vi "test-FIX Helper Dialog.vi"() -> ()   [LabVIEW 2017]
panel:
  in  "Bottom Text":string="Communicable State Machine(CSM) v2024.11.28.152636        "
  out "2D Picture":picture
  out "Progress Bar":i32(slide) scale=0.0..100.0
  in  "path to PNG file":path
  # "图片尺寸=768 x 432"
  # "VI 宽度=768-24=744"
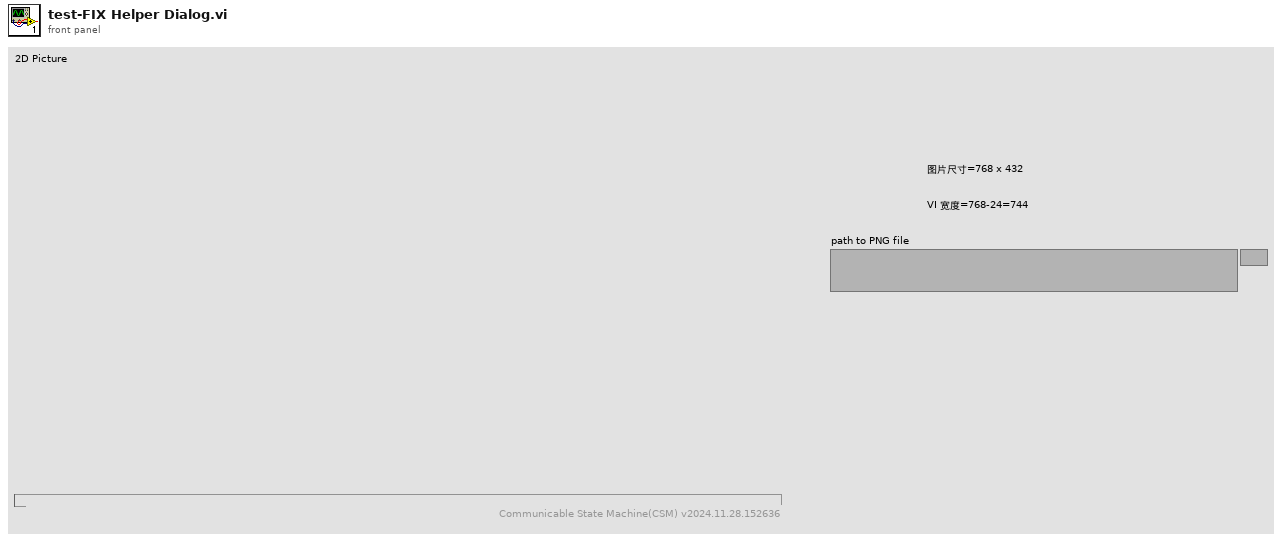
[diagram p1: front panel]
types:
  T1 = typedef "imagedata.ctl" = cluster{"image type":i32, "image depth":i32, "image":u8[], "mask":u8[], "colors":u32[], "Rectangle":cluster{"left":i16, "top":i16, "right":i16, "bottom":i16}}
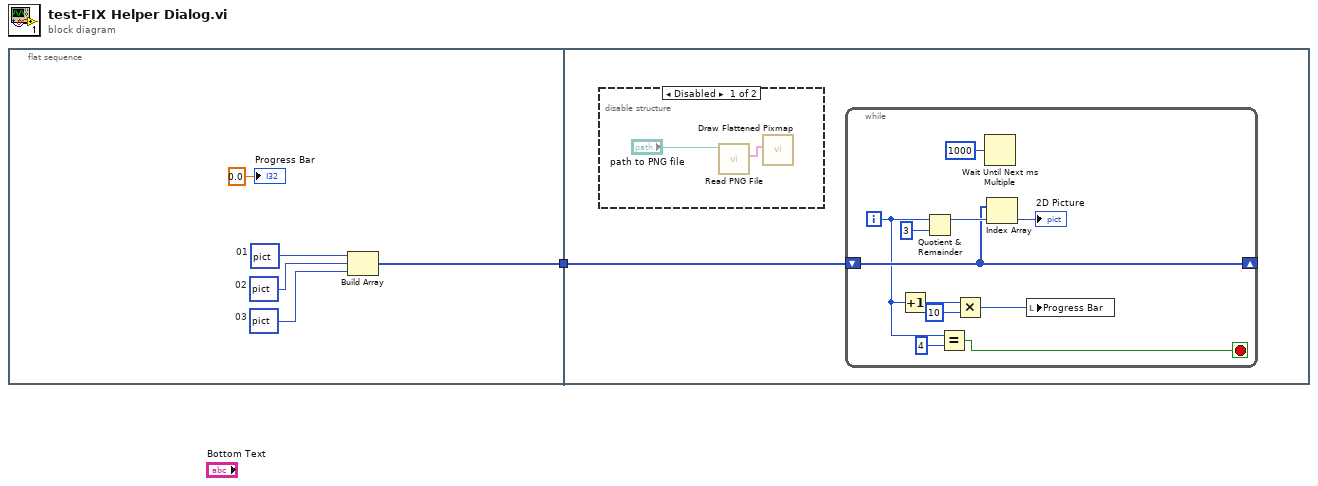
[diagram p0: block diagram]
diagram:
  n1 = flat-sequence {
    tunnel: [w3] -> w1
    tunnel: w1 -> [w7]
    frame #0 {
      w4 = picture bytes[1036830]  # 03
      w5 = picture bytes[1036830]  # 02
      w6 = picture bytes[1036830]  # 01
      n2 = Build Array(w6, w5, w4) -> (w3:picture[])
      "Progress Bar" <- 0.0 ("Progress Bar")
    }
    frame #1 {
      n3 = disable-structure shown="Disabled" {
        frame Disabled {
          n4 = call <vilib>:"Read PNG File.vi"("path to PNG file"="path to PNG file") -> ("image data"=w20:T1)  [unwired: 8 in, 2 out]
          n5 = call <vilib>:"Draw Flattened Pixmap.vi"("image data"=w20) -> ()  [unwired: 8 in, 1 out]
        }
        frame Enabled {
        }
      }
      n6 = while {
        shift-right: [w16] -> _
        shift-left: w7 -> [w16]
        i -> [w10]
        stop <- w8 stop-if-true
        n7 = Increment(x=w10) -> (x+1=w12:i32)
        n8 = Quotient & Remainder(x=w10, y=3) -> (x-y*floor(x/y)=w17:i32)  [unwired: 1 out]
        n9 = Equal?(x=w10, y=4) -> (x = y?=w8:bool)
        n10 = Multiply(x=w12, y=10) -> (x*y=w13:i32)
        n11 = Wait Until Next ms Multiple(millisecond multiple=u32 1000) -> ()  [unwired: 1 out]
        n12 = Index Array(array=w16, index=w17) -> (element=→"2D Picture":picture)
        n13 = local write "Progress Bar"(w13) -> ()
      }
    }
  }
